vi "TWC.vi"(0 "System no.":i32=1 min=1 max=4 step=1, 5 "error in":errorcluster) -> (19 "error out":errorcluster)   [LabVIEW 2020]
doc: "Clears the trigger settings for the waveform."
panel:
  # "Clears the trigger wave settings for the waveform."
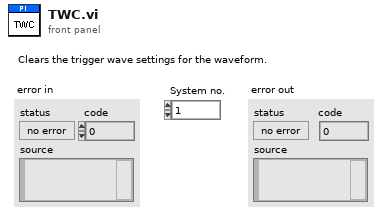
[diagram p1: front panel]
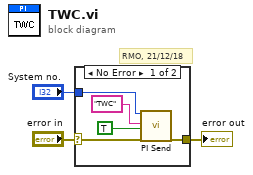
[diagram p0: block diagram]
diagram:
  # "RMO, 21/12/18"
  n1 = case shown="No Error" "error in" {
    selector: "error in" -> [w4 w9]
    tunnel: "System no." -> [w6 _]
    tunnel: [w5 w9] -> w2
    frame No Error {
      n2 = call "PI Send.vi"("System no."=w6, "String to send"="TWC", "Attach termination char.?"=TRUE ("Attach Linefeed?"), "error in"=w4) -> ("error out"=w5:errorcluster)  [unwired: 2 in, 13 out]
    }
    frame Error {
    }
  }
  "error out" <- w2
